vi "DAQ-AI Mean Value.vi"(8 "Cluster":T1, 11 "data":dbl[][](array[numeric]) format="%0.2f") -> (3 "Analoge Input":dbl[](array[numeric]))   [LabVIEW 2015]
uses:
  <vilib>/Analysis/baseanly.llb/Mean (DBL).vi
  Galobal variable_TI.vi
  <vilib>/Analysis/NI_AALBase.lvlib
  <vilib>/ptbypt/NI_PtbyPt.lvlib
panel:
  out "Waveform Chart":dbl(graph)
  out "AI_as DI":bool[](array[boolean])
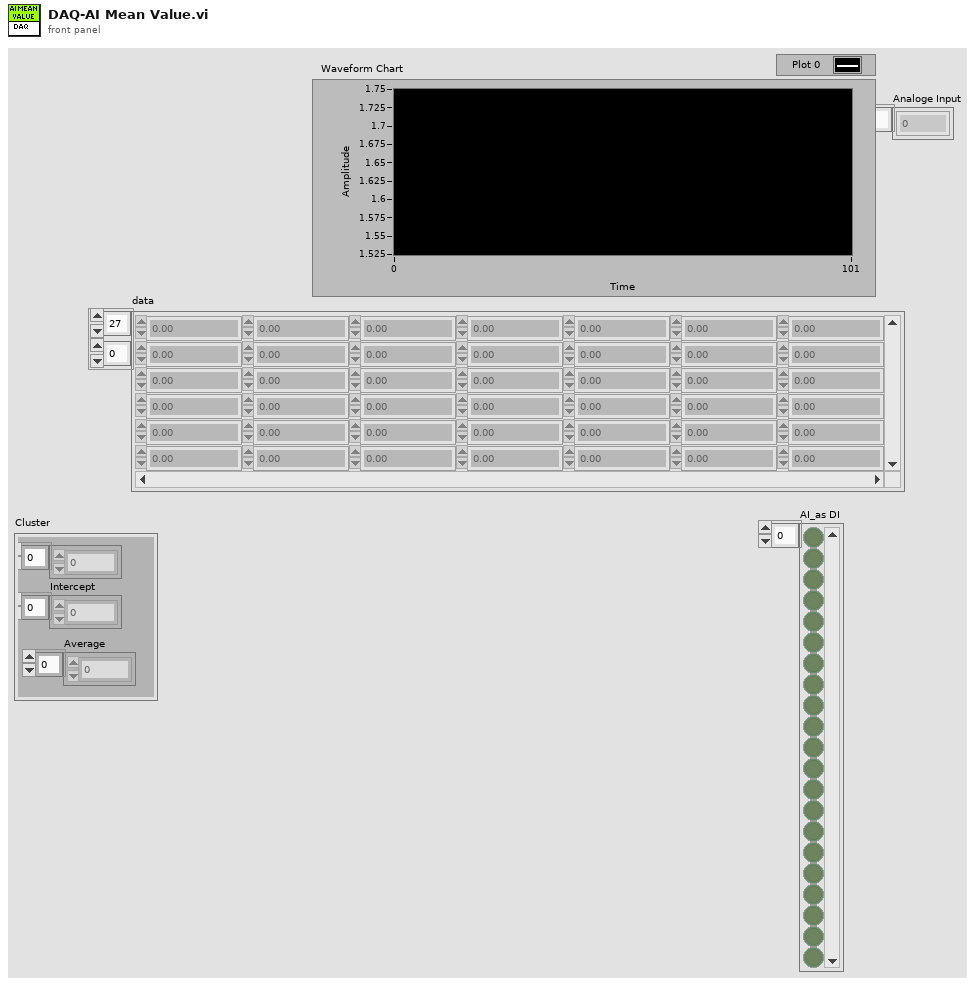
[diagram p1: front panel]
types:
  T1 = cluster{"Slop":dbl[], "Intercept":dbl[], "Average ":i16[]}
  T2 = cluster{"IL Sensor1_AI04":dbl, "IL Sensor1_AI05":dbl, "IL Sensor1_AI04":bool, "IL Sensor1_AI05":bool}
  T3 = cluster{"ILSensormax_1":dbl, "ILSensormin_1":dbl, "ILSensormax _2":dbl, "ILSensormin_2":dbl}
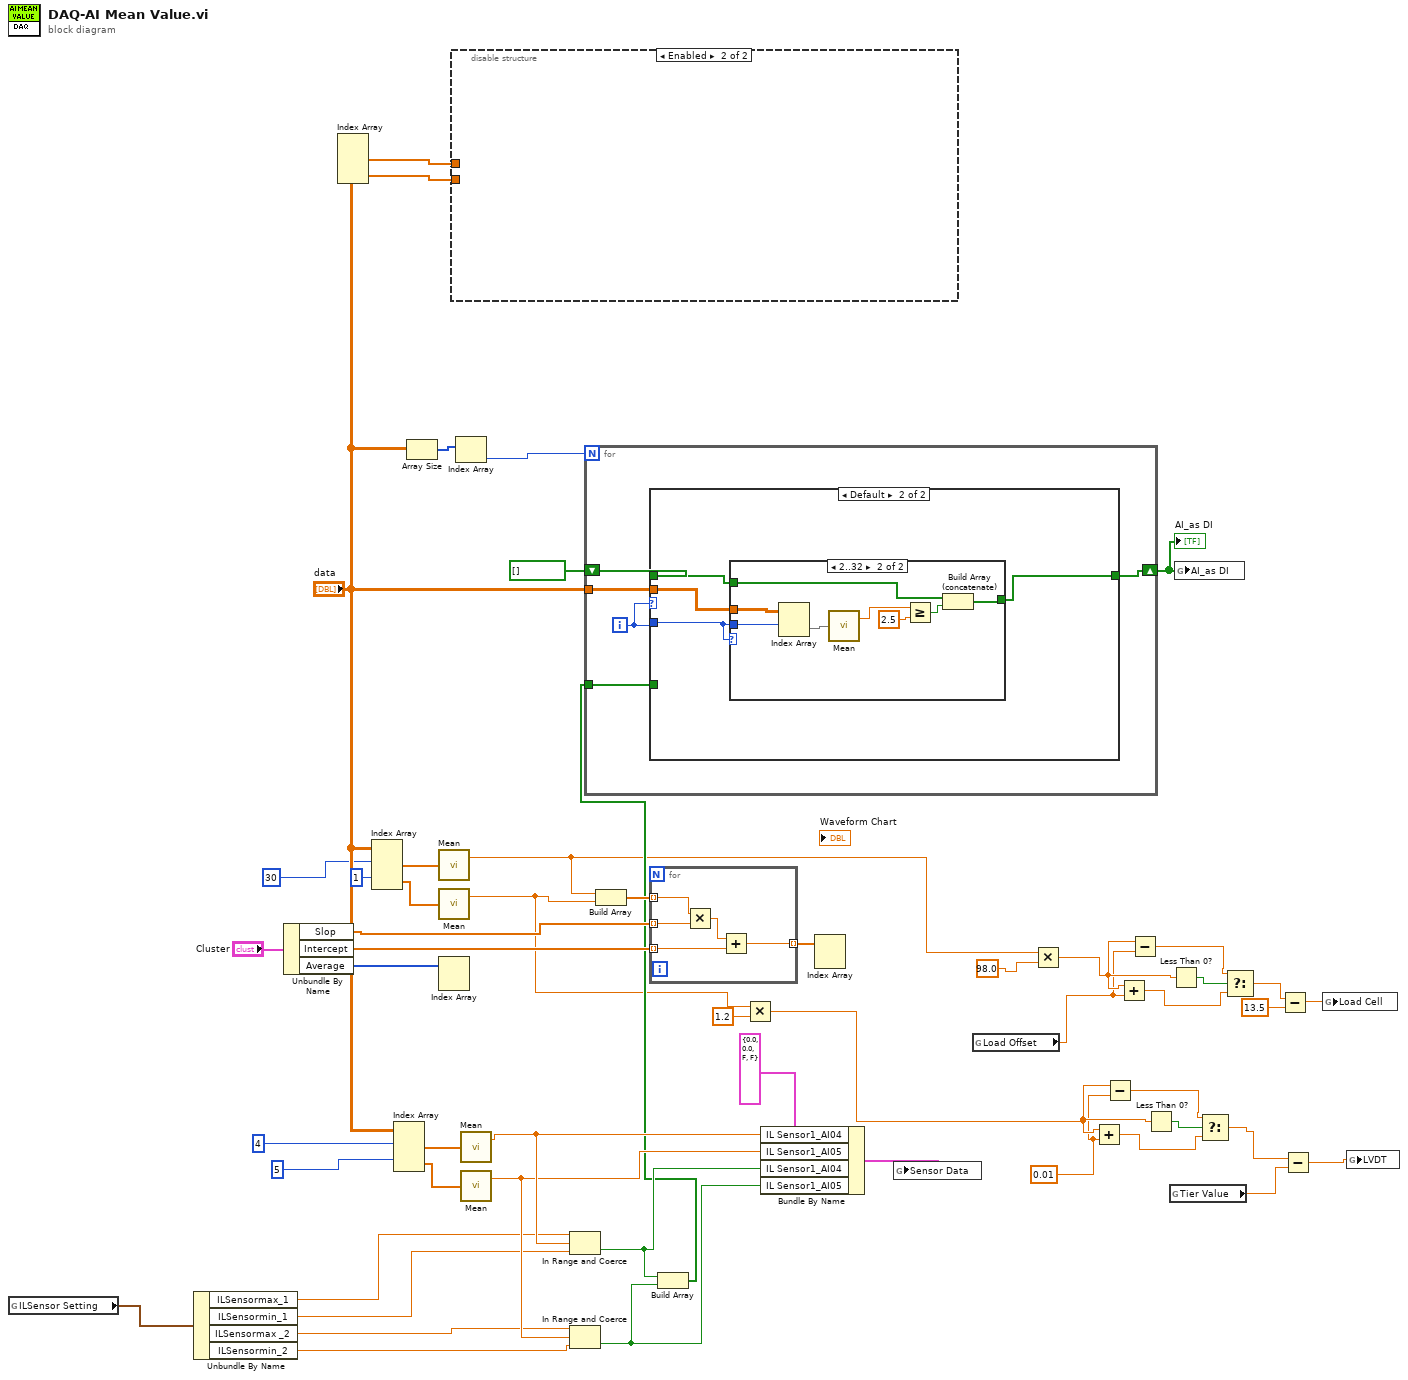
[diagram p0: block diagram]
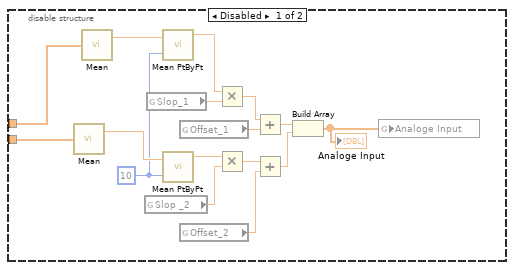
[diagram p2: hidden frame]
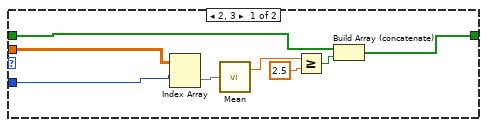
[diagram p3: hidden frame]
diagram:
  w7 = 0.01 ("Tier Value")
  n1 = global read "Galobal variable_TI.vi" "ILSensor Setting"() -> (w31:T3)
  n2 = Unbundle By Name(w31) -> ("ILSensormax_1"=w30:dbl, "ILSensormin_1"=w29:dbl, "ILSensormax _2"=w28:dbl, "ILSensormin_2"=w27:dbl)
  n3 = Unbundle By Name("Cluster") -> ("Slop"=w42:dbl[], "Intercept"=w41:dbl[], "Average"=w40:i16[])
  n4 = Index Array(array="data") -> (element #1=w50:dbl[], element #2=w53:dbl[])  [unwired: 4 in]
  n5 = Index Array(array="data", index (row) #1=30 ("index (row)"), index (row) #2=1 ("index (row)")) -> (element #1=w44:dbl[], element #2=w43:dbl[])  [unwired: 2 in]
  n6 = Index Array(array="data", index (row) #1=4 ("index (row)"), index (row) #2=5) -> (element #1=w38:dbl[], element #2=w39:dbl[])  [unwired: 2 in]
  n7 = Array Size(array="data") -> (size(s)=w52:i32[])
  n8 = call-poly <vilib>:"Mean.vi"("X"=w44) -> ("mean"=w14:dbl)  [unwired: 1 out]
  n9 = call-poly <vilib>:"Mean.vi"("X"=w43) -> ("mean"=w13:dbl)  [unwired: 1 out]
  n10 = Index Array(array=w40) -> ()  [unwired: 2 in, 2 out]
  n11 = disable-structure shown="Enabled" {
    disable-tunnel: w53 -> [w69 _]
    disable-tunnel: w50 -> [w66 _]
    frame Disabled {
      w65 = 10 ("sample length")
      n12 = call-poly <vilib>:"Mean.vi"("X"=w69) -> ("mean"=w67:dbl)  [unwired: 1 out]
      n13 = call-poly <vilib>:"Mean.vi"("X"=w66) -> ("mean"=w68:dbl)  [unwired: 1 out]
      n14 = global read "Galobal variable_TI.vi" "Slop _2"() -> (w57:dbl)
      n15 = global read "Galobal variable_TI.vi" "Slop_1"() -> (w62:dbl)
      n16 = call <vilib>:"Mean PtByPt.vi"("x"=w68, "sample length"=w65) -> ("mean"=w63:dbl)  [unwired: 2 in, 1 out]
      n17 = call <vilib>:"Mean PtByPt.vi"("x"=w67, "sample length"=w65) -> ("mean"=w58:dbl)  [unwired: 2 in, 1 out]
      n18 = global read "Galobal variable_TI.vi" "Offset_1"() -> (w60:dbl)
      n19 = global read "Galobal variable_TI.vi" "Offset_2"() -> (w56:dbl)
      n20 = Multiply(x=w63, y=w62) -> (x*y=w61:dbl)
      n21 = Multiply(x=w58, y=w57) -> (x*y=w59:dbl)
      n22 = Add(x=w61, y=w60) -> (x+y=w55:dbl)
      n23 = Add(x=w59, y=w56) -> (x+y=w54:dbl)
      n24 = Build Array(w55, w54) -> (w64:dbl[])
      "Analoge Input" <- w64
      n25 = global write "Galobal variable_TI.vi" "Analoge Input"(w64) -> ()
    }
    frame Enabled {
    }
  }
  n26 = Index Array(array=w52) -> (element=w49:i32)  [unwired: 1 in]
  n27 = call-poly <vilib>:"Mean.vi"("X"=w38) -> ("mean"=w33:dbl)  [unwired: 1 out]
  n28 = call-poly <vilib>:"Mean.vi"("X"=w39) -> ("mean"=w32:dbl)  [unwired: 1 out]
  n29 = In Range and Coerce(upper limit=w30, x=w33, lower limit=w29) -> (In Range?=w25:bool)  [unwired: 1 out]
  n30 = In Range and Coerce(upper limit=w28, x=w32, lower limit=w27) -> (In Range?=w24:bool)  [unwired: 1 out]
  n31 = Build Array(w14, w13) -> (w45:dbl[])
  n32 = for {
    tunnel: w42 -> [w74] mode=indexing
    tunnel: w41 -> [w72] mode=indexing
    tunnel: w45 -> [w70] mode=indexing
    tunnel: [w71] -> w46 mode=indexing
    n33 = Multiply(x=w70, y=w74) -> (x*y=w73:dbl)
    n34 = Add(x=w73, y=w72) -> (x+y=w71:dbl)
  }
  n35 = Build Array(w25, w24) -> (w23:bool[])
  n36 = for {
    N: w49 -> [_]
    tunnel: "data" -> [w79]
    shift-right: [w77] -> w48
    shift-left: bool[] [] -> [w76]
    tunnel: w23 -> [w75]
    i -> [w78]
    n37 = case shown="Default" w78 {
      tunnel: w79 -> [w82 w90]
      tunnel: w78 -> [w81 w89]
      tunnel: [w80 w88] -> w77
      tunnel: w76 -> [w83 w91]
      tunnel: w75 -> [_ _]
      frame 2, 3 {
        n38 = Index Array(array=w82, index (row)=w81) -> (element=w85:dbl[])  [unwired: 1 in]
        n39 = call-poly <vilib>:"Mean.vi"("X"=w85) -> ("mean"=w84:dbl)  [unwired: 1 out]
        n40 = Greater Or Equal?(x=w84, y=2.5) -> (x >= y?=w86:bool)
        n41 = Build Array (concatenate)(w83, w86) -> (w80:bool[])
      }
      frame Default {
        n42 = case shown="2..32" w89 {
          tunnel: w90 -> [_ w96]
          tunnel: w91 -> [w92 w95]
          tunnel: [w92 w94] -> w88
          tunnel: w89 -> [_ w93]
          frame 0, Default {
          }
          frame 2..32 {
            n43 = Index Array(array=w96, index (row)=w93) -> (element=w98:dbl[])  [unwired: 1 in]
            n44 = call-poly <vilib>:"Mean.vi"("X"=w98) -> ("mean"=w97:dbl)  [unwired: 1 out]
            n45 = Greater Or Equal?(x=w97, y=2.5) -> (x >= y?=w99:bool)
            n46 = Build Array (concatenate)(w95, w99) -> (w94:bool[])
          }
        }
      }
    }
  }
  "AI_as DI" <- w48
  n47 = Multiply(x=w13, y=1.2) -> (x*y=w8:dbl)
  n48 = Bundle By Name(cluster=T2 {"IL Sensor1_AI04"=0.0, "IL Sensor1_AI05"=0.0, "IL Sensor1_AI04"=FALSE, "IL Sensor1_AI05"=FALSE} ("Sensor Data 2"), "IL Sensor1_AI04"=w33, "IL Sensor1_AI05"=w32, "IL Sensor1_AI04"=w25, "IL Sensor1_AI05"=w24) -> (w26:T2)
  n49 = Index Array(array=w46) -> ()  [unwired: 2 in, 2 out]
  n50 = global write "Galobal variable_TI.vi" "Sensor Data"(w26) -> ()
  n51 = global read "Galobal variable_TI.vi" "Load Offset"() -> (w15:dbl)
  n52 = Multiply(x=w14, y=98.0) -> (x*y=w19:dbl)
  n53 = Add(x=w8, y=w7) -> (x+y=w11:dbl)
  n54 = Subtract(x=w8, y=w7) -> (x-y=w10:dbl)
  n55 = Add(x=w19, y=w15) -> (x+y=w17:dbl)
  n56 = Subtract(x=w19, y=w15) -> (x-y=w18:dbl)
  n57 = Less Than 0?(x=w8) -> (x < 0?=w9:bool)
  n58 = global read "Galobal variable_TI.vi" "Tier Value"() -> (w5:dbl)
  n59 = Less Than 0?(x=w19) -> (x < 0?=w20:bool)
  n60 = global write "Galobal variable_TI.vi" "AI_as DI"(w48) -> ()
  n61 = Select(t=w10, s=w9, f=w11) -> (s? t:f=w6:dbl)
  n62 = Select(t=w18, s=w20, f=w17) -> (s? t:f=w3:dbl)
  n63 = Subtract(x=w3, y=13.5) -> (x-y=w1:dbl)
  n64 = Subtract(x=w6, y=w5) -> (x-y=w4:dbl)
  n65 = global write "Galobal variable_TI.vi" "Load Cell"(w1) -> ()
  n66 = global write "Galobal variable_TI.vi" "LVDT"(w4) -> ()
